vi "Get Movie Settings.vi"(8 "error in (no error)":errorcluster, 11 "Protocol in":refnum<class "Protocol.lvclass">) -> (0 "error out":errorcluster, 2 "Movie Settings Array":T1[](array[typedef]) {"Camera Settings"."Exposure Time (ms)" min=1.0 max=10000.0 step=1.0}, 3 "Protocol out":refnum<class "Protocol.lvclass">)   [LabVIEW 2023, in "Automation.lvlib" / "Protocol.lvclass"]
uses:
  Protocol.lvclass
  Resources/Type Defs/Movie Settings.ctl
  Resources/Type Defs/Camera Settings.ctl
  Protocol.lvclass/Protocol.ctl
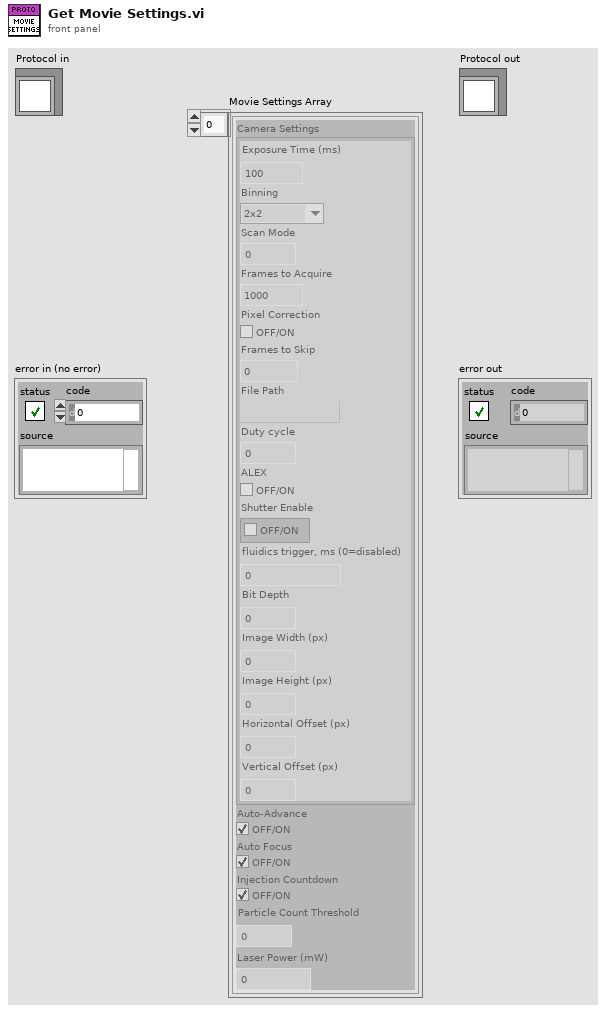
[diagram p1: front panel]
types:
  T1 = typedef "Movie Settings.ctl" = cluster{"Camera Settings":T2, "Auto-Advance":bool, "Auto Focus":bool, "Injection Countdown":bool, "Particle Count Threshold":i32, "Laser Power (mW)":u32}
  T2 = typedef "Camera Settings.ctl" = cluster{"Exposure Time (ms)":dbl, "Binning":enum16{"1x1", "2x2", "4x4"}, "Scan Mode":i32, "Frames to Acquire":dbl, "Pixel Correction":bool, "Frames to Skip":u32, "File Path":path, "Duty cycle":dbl, "ALEX":bool, "Shutter Enable":bool[], "fluidics trigger, ms (0=disabled)":dbl, "Bit Depth":u16, "Image Width (px)":u16, "Image Height (px)":u16, "Horizontal Offset (px)":u16, "Vertical Offset (px)":u16}
  T3 = typedef "Movie Series.ctl" = cluster{"Fields":i32, "Lanes":i32, "Acquisition type":T4, "Sweep":T5}
  T4 = typedef "Movie auto-numbering.ctl" = enum16{"Single movie", "Movie series", "Multi-lane series", "Sweep Parameter"}
  T5 = typedef "Param Sweep.ctl" = cluster{"Parameter":enum16{"Laser Power (mW)", "Exposure Time (ms)"}, "Values":u32[], "Repeats":u32}
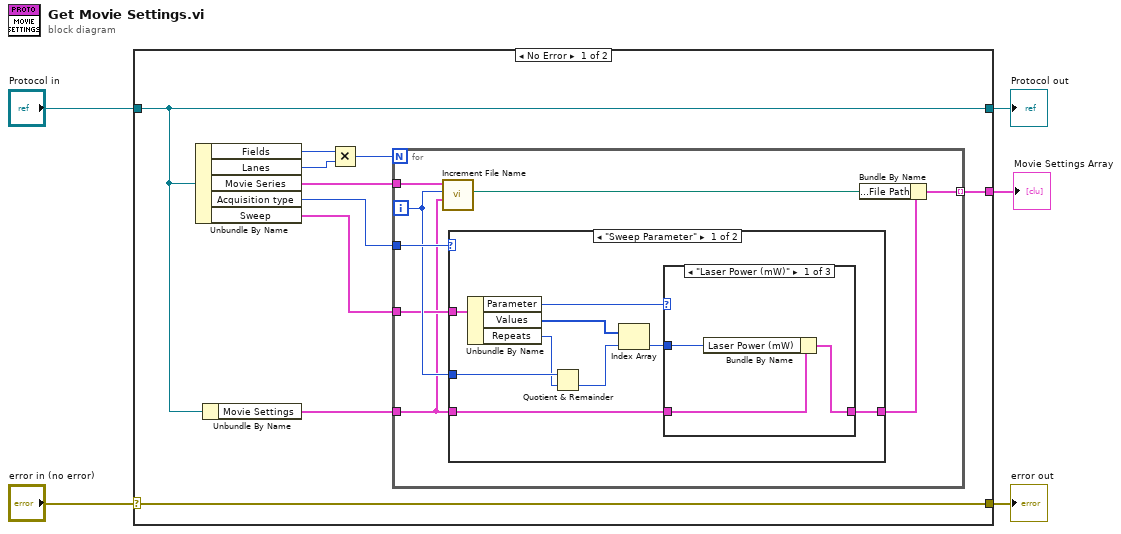
[diagram p0: block diagram]
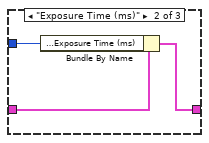
[diagram p2: hidden frame]
diagram:
  n1 = case shown="No Error" "error in (no error)" {
    selector: "error in (no error)" -> [w15 w42]
    tunnel: [w15 w42] -> w4
    tunnel: [w7 w41] -> w2
    tunnel: "Protocol in" -> [w7 w41]
    tunnel: [w14 _] -> w1
    frame No Error {
      n2 = Unbundle By Name(w7) -> ("Fields"=w12:i32, "Lanes"=w11:i32, "Movie Series"=w13:T3, "Acquisition type"=w9:T4, "Sweep"=w8:T5)
      n3 = Unbundle By Name(w7) -> ("Movie Settings"=w6:T1)
      n4 = Multiply(x=w12, y=w11) -> (x*y=w10:i32)
      n5 = for {
        N: w10 -> [_]
        tunnel: [w23] -> w14 mode=indexing
        tunnel: w13 -> [w22]
        tunnel: w9 -> [w20]
        tunnel: w6 -> [w16]
        tunnel: w8 -> [w17]
        i -> [w18]
        n6 = call "Increment File Name.vi"("Movie Settings"=w16, "Movie Index"=w18, "Movie Series In"=w22) -> ("FIle Path Out"=w21:path)  [unwired: 8 in]
        n7 = case shown="\"Sweep Parameter\"" w20 {
          tunnel: w16 -> [w31 w40]
          tunnel: [w29 w40] -> w19
          tunnel: w18 -> [w26 _]
          tunnel: w17 -> [w32 _]
          frame "Sweep Parameter" {
            n8 = Unbundle By Name(w32) -> ("Parameter"=w30:enum16{"Laser Power (mW)", "Exposure Time (ms)"}, "Values"=w28:u32[], "Repeats"=w25:u32)
            n9 = Quotient & Remainder(x=w26, y=w25) -> (floor(x/y)=w24:u32)  [unwired: 1 out]
            n10 = Index Array(array=w28, index=w24) -> (element=w27:u32)
            n11 = case shown="\"Laser Power (mW)\"" w30 {
              tunnel: w31 -> [w34 w37 w39]
              tunnel: [w35 w38 w39] -> w29
              tunnel: w27 -> [w33 w36 _]
              frame "Laser Power (mW)" {
                n12 = Bundle By Name(cluster=w34, "Laser Power (mW)"=w33) -> (w35:T1)
              }
              frame "Exposure Time (ms)" {
                n13 = Bundle By Name(cluster=w37, "Camera Settings.Exposure Time (ms)"=w36) -> (w38:T1)
              }
              frame Default {
              }
            }
          }
          frame Default {
          }
        }
        n14 = Bundle By Name(cluster=w19, "Camera Settings.File Path"=w21) -> (w23:T1)
      }
    }
    frame Error {
    }
  }
  "error out" <- w4
  "Protocol out" <- w2
  "Movie Settings Array" <- w1
